vi "GPinApp.vi"() -> ()   [LabVIEW 2010]
panel:
  out "GP In State":bool
  in  "stop":bool
  in  "ICImagingControl":refnum<k7>(container)
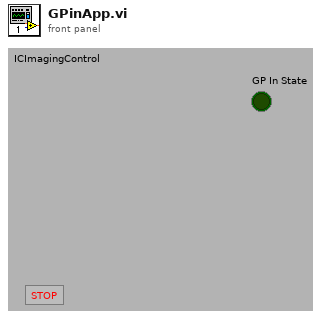
[diagram p1: front panel]
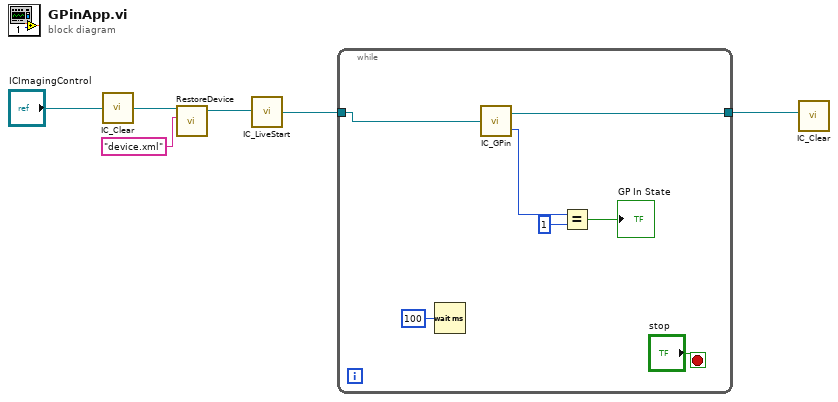
[diagram p0: block diagram]
diagram:
  n1 = call <userlib>:"IC_Clear.vi"("ICImagingControl 2"="ICImagingControl") -> ("ICImagingControl"=w3:refnum<k7>)
  n2 = call <userlib>:"RestoreDevice.vi"("Filename"="device.xml", "ICImagingControl"=w3) -> ("ICImagingControl 2"=w2:refnum<k7>)  [unwired: 2 in, 2 out]
  n3 = call <userlib>:"IC_LiveStart.vi"("ICImagingControl 3"=w2) -> ("ICImagingControl 2"=w5:refnum<k7>)
  n4 = while {
    tunnel: w5 -> [w12]
    tunnel: [w11] -> w4
    stop <- "stop" stop-if-true
    n5 = Wait (ms)(milliseconds to wait=u32 100) -> ()  [unwired: 1 out]
    n6 = call "IC_GPin.vi"("ICImagingControl 3"=w12) -> ("ICImagingControl 2"=w11:refnum<k7>, "GP In"=w9:i32)
    n7 = Equal?(x=w9, y=1) -> (x = y?=→"GP In State":bool)
  }
  n8 = call <userlib>:"IC_Clear.vi"("ICImagingControl 2"=w4) -> ()  [unwired: 1 out]
